vi "Write Limit.vi"(8 "error in (no error)":errorcluster, 10 "Limit":string[][](array[string]), 11 "TestEngine in":refnum<class "TestEngine.lvclass">) -> (0 "error out":errorcluster, 3 "TestEngine out":refnum<class "TestEngine.lvclass">)   [LabVIEW 2019, in "TestEngine.lvlib" / "TestEngine.lvclass"]
uses:
  TestEngine.lvclass
  TestEngine.lvclass/TestEngine.ctl
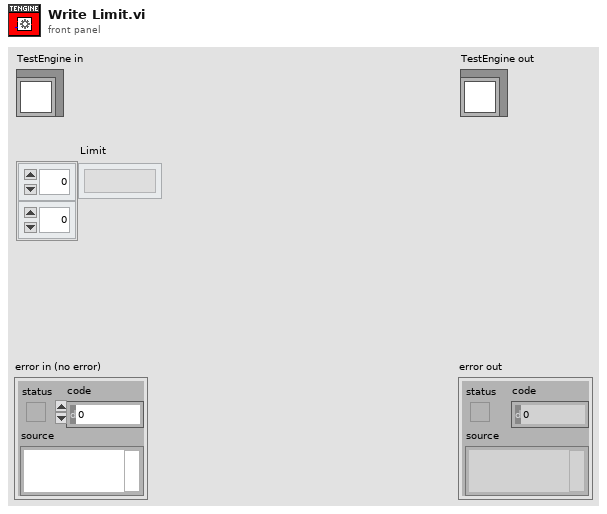
[diagram p1: front panel]
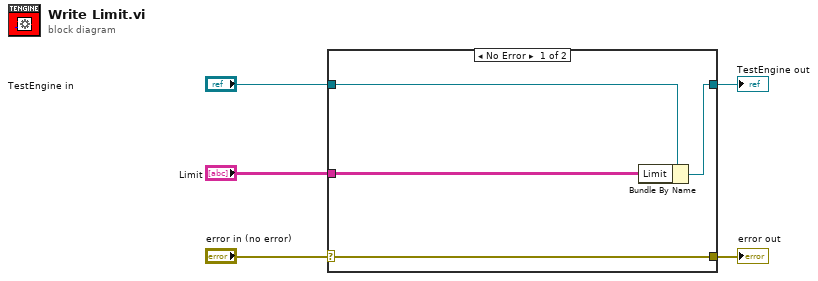
[diagram p0: block diagram]
diagram:
  n1 = case shown="No Error" "error in (no error)" {
    selector: "error in (no error)" -> [w9 w10]
    tunnel: [w9 w10] -> w4
    tunnel: [w7 w11] -> w2
    tunnel: "TestEngine in" -> [w8 w11]
    tunnel: "Limit" -> [w6 _]
    frame No Error {
      n2 = Bundle By Name(cluster=w8, "Limit"=w6) -> (w7:refnum<class "TestEngine.lvclass">)
    }
    frame Error {
    }
  }
  "error out" <- w4
  "TestEngine out" <- w2
